vi "find variables.vi"() -> ()   [LabVIEW 2017]
panel:
  out "outputvalue":dbl format="%#_13g"
  out "indexno":i32
  in  "varin":string="Psuc"
  in  "numarray":dbl[](array[numeric])
  in  "varnames":string[](array[string])
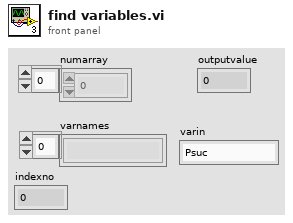
[diagram p1: front panel]
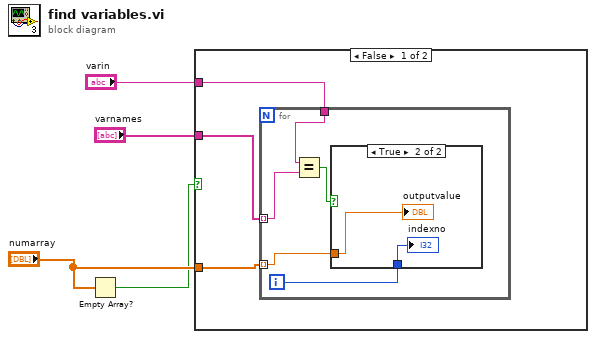
[diagram p0: block diagram]
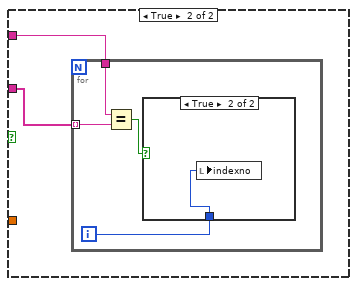
[diagram p3: hidden frame]
diagram:
  n1 = Empty Array?(array="numarray") -> (empty?=w1:bool)
  n2 = case shown="False" w1 {
    tunnel: "varin" -> [w7 w15]
    tunnel: "varnames" -> [w6 w16]
    tunnel: "numarray" -> [w5 _]
    frame False {
      n3 = for {
        tunnel: w5 -> [w9] mode=indexing
        tunnel: w6 -> [w12] mode=indexing
        tunnel: w7 -> [w11]
        i -> [w8]
        n4 = Equal?(x=w11, y=w12) -> (x = y?=w10:bool)
        n5 = case shown="True" w10 {
          tunnel: w9 -> [_ w14]
          tunnel: w8 -> [_ w13]
          frame False {
          }
          frame True {
            "outputvalue" <- w14
            "indexno" <- w13
          }
        }
      }
    }
    frame True {
      n6 = for {
        tunnel: w16 -> [w18] mode=indexing
        tunnel: w15 -> [w17]
        i -> [w19]
        n7 = Equal?(x=w17, y=w18) -> (x = y?=w20:bool)
        n8 = case shown="True" w20 {
          tunnel: w19 -> [_ w21]
          frame False {
          }
          frame True {
            n9 = local write "indexno"(w21) -> ()
          }
        }
      }
    }
  }
